vi "Validate Sequence JSON.vi"(7 "Fallback Name":string, 8 "error in (no error)":errorcluster, 10 "JSON":string) -> (0 "error out":errorcluster)   [LabVIEW 2023, in "VolatusSeq.lvlib" / "Sequence Validation.lvclass"]
uses:
  Sequence Validation.lvclass
  Sequence Validation.lvclass/Sequence Validation.ctl
  VolatusErrorUtilities/MultiErrors/MultiErrors.lvclass
  Sequence Config/Sequence Config.lvclass
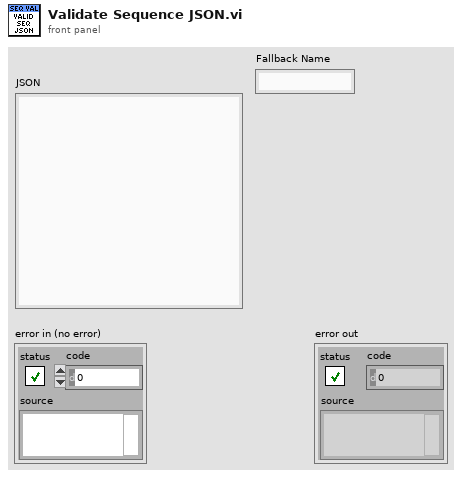
[diagram p1: front panel]
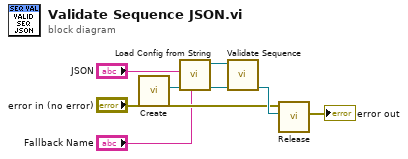
[diagram p0: block diagram]
diagram:
  n1 = call "Create.vi"() -> ("MultiErrors out"=w8:refnum<class "MultiErrors.lvclass">)  [unwired: 11 in]
  n2 = call "Load Config from String.vi"("Fallback Name"="Fallback Name", "error in (no error)"=w8, "JSON"="JSON") -> ("error out"=w7:refnum<class "MultiErrors.lvclass">, "Sequence Config"=w6:refnum<class "Sequence Config.lvclass">)  [unwired: 7 in]
  n3 = call "Validate Sequence.vi"("error in (no error)"=w7, "Sequence Config in"=w6) -> ("error out"=w4:refnum<class "MultiErrors.lvclass">)  [unwired: 8 in, 1 out]
  n4 = call "Release.vi"("MultiErrors in"=w4, "Upstream Error (None)"="error in (no error)") -> ("error out"=→"error out":errorcluster)  [unwired: 9 in]
